vi "Drive Base - GRIP Set.vi"(8 "error in (no error)":errorcluster, 11 "Target GRIP Area":dbl) -> (0 "error out":errorcluster)   [LabVIEW 2015]
uses:
  Drive Base Mode.ctl
  Drive Base - Controlled Mode - TypeDef.ctl
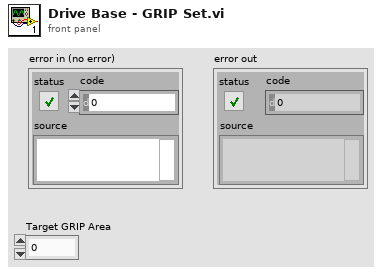
[diagram p1: front panel]
types:
  T1 = typedef "Drive Base - Controlled Mode - TypeDef.ctl" = cluster{"Drive Base Mode":T2, "Arcade":cluster{"y":dbl, "x":dbl}, "Tank":cluster{"Left":dbl, "Right":dbl}, "Target Encoder Value":cluster{"Left":dbl, "Right":dbl}, "Target IMU Angle":dbl, "Distance":dbl, "Target GRIP Area":dbl}
  T2 = typedef "Drive Base Mode.ctl" = enum16{"Off", "Controlled - Arcade", "Controlled - Tank", "Braked", "GRIP", "Encoder", "IMU", "Distance"}
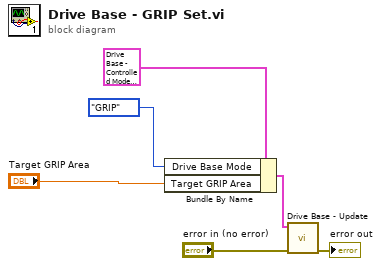
[diagram p0: block diagram]
diagram:
  n1 = Bundle By Name(cluster=T1 {"Drive Base Mode"=enum."Off", "Arcade"={"y"=0.0, "x"=0.0}, "Tank"={"Left"=0.0, "Right"=0.0}, "Target Encoder Value"={"Left"=0.0, "Right"=0.0}, "Target IMU Angle"=0.0, "Distance"=0.0, "Target GRIP Area"=0.0}, "Drive Base Mode"=Drive_Base_Mode."GRIP", "Target GRIP Area"="Target GRIP Area") -> (w5:T1)
  n2 = call "Drive Base - Update.vi"("error in (no error)"="error in (no error)", "Drive Base Notifier"=w5) -> ("error out"=→"error out":errorcluster)  [unwired: 9 in]
